vi "niDTS WLAN UTIL Freq to Channel.vi"(6 "secondary factor":i32(ring)=-1 items=["-1"=-1, "1"=1, "0"=0], 8 "error in":errorcluster, 9 "channel starting factor":dbl=10000.0, 10 "CH BW":T1=enum."160 MHz", 11 "Center Frequency":dbl) -> (0 "error out":errorcluster, 3 "Channel":u32)   [LabVIEW 2015, in "niDTS WLAN.lvlib"]
uses:
  niDTS WLAN.lvlib
  Includes/niDTS WLAN INC CH BW.ctl
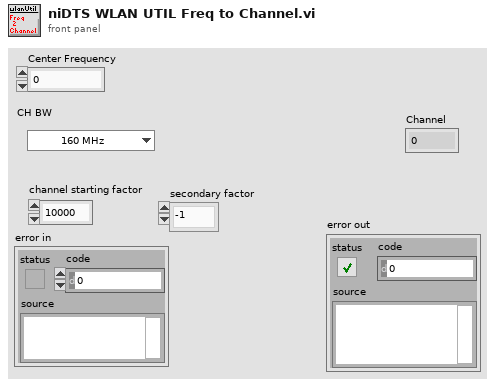
[diagram p1: front panel]
types:
  T1 = typedef "niDTS WLAN.lvlib/niDTS WLAN INC CH BW.ctl" = enum16{"20 MHz", "40 MHz", "80 MHz", "160 MHz"}
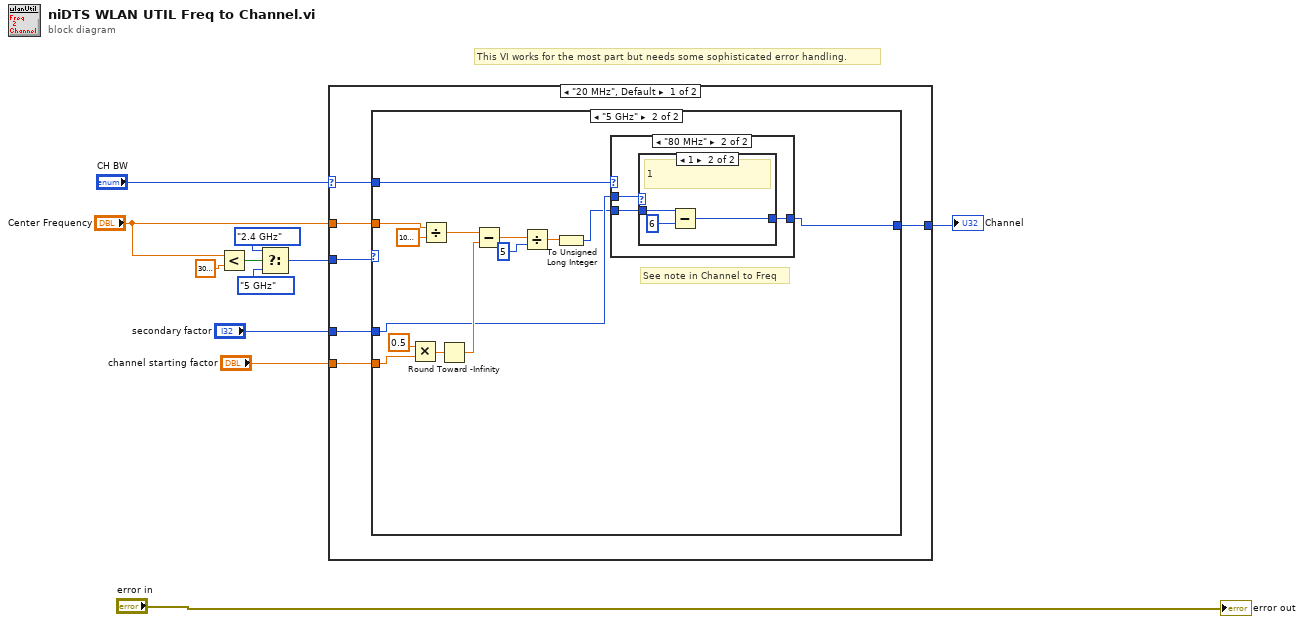
[diagram p0: block diagram]
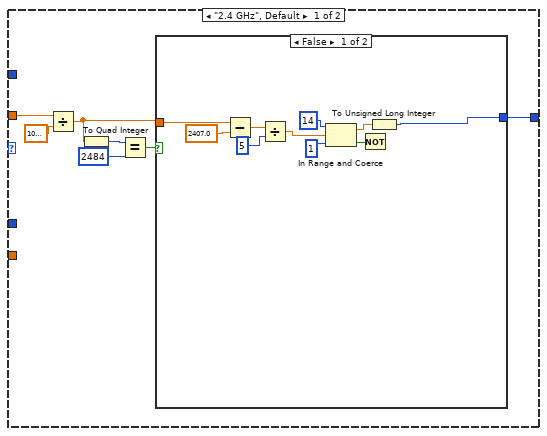
[diagram p2: hidden frame]
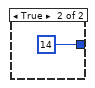
[diagram p3: hidden frame]
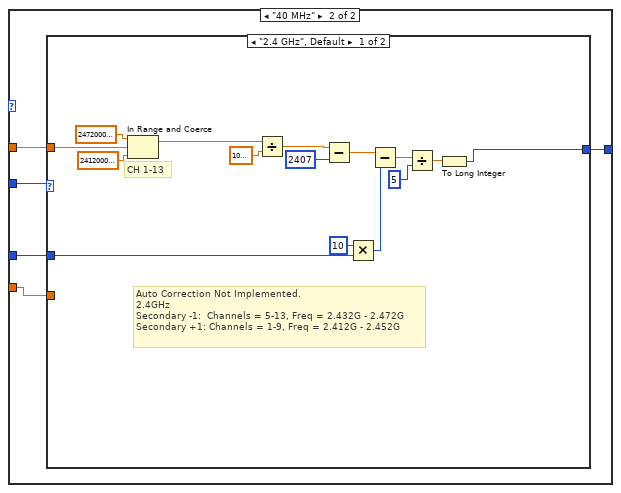
[diagram p6: hidden frame]
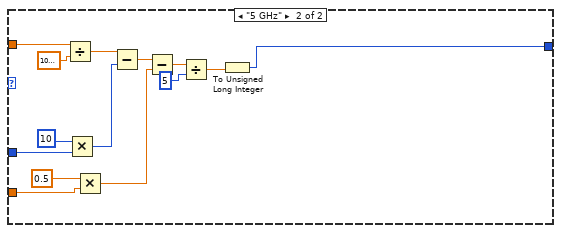
[diagram p7: hidden frame]
diagram:
  # "This VI works for the most part but needs some sophisticated error handling."
  n1 = Less?(x="Center Frequency", y=3000000000.0) -> (x < y?=w8:bool)
  n2 = Select(t=enum16{"2.4 GHz", "5 GHz"}."2.4 GHz" ("frequency band"), s=w8, f=enum16{"2.4 GHz", "5 GHz"}."5 GHz" ("frequency band")) -> (s? t:f=w7:enum16{"2.4 GHz", "5 GHz"})
  n3 = case shown="\"20 MHz\", Default" "CH BW" {
    selector: "CH BW" -> [w13 _]
    tunnel: w7 -> [w17 w62]
    tunnel: "Center Frequency" -> [w16 w61]
    tunnel: [w15 w59] -> w5
    tunnel: "secondary factor" -> [w12 w60]
    tunnel: "channel starting factor" -> [w14 w58]
    frame "20 MHz", Default {
      n4 = case shown="\"5 GHz\"" w17 {
        tunnel: w16 -> [w18 w40]
        tunnel: [w20 w36] -> w15
        tunnel: w14 -> [_ w45]
        tunnel: w13 -> [_ w39]
        tunnel: w12 -> [_ w38]
        frame "2.4 GHz", Default {
          n5 = Divide(x=w18, y=1000000.0) -> (x/y=w19:dbl)
          n6 = To Quad Integer(1:w19) -> (0:w23:i64)
          n7 = Equal?(x=w23, y=i64 2484) -> (x = y?=w21:bool)
          n8 = case shown="False" w21 {
            tunnel: [w25 u32 14 ("Channel")] -> w20
            tunnel: w19 -> [w33 _]
            frame False {
              n9 = Subtract(x=w33, y=2407.0 ("x")) -> (x-y=w32:dbl)
              n10 = Divide(x=w32, y=5) -> (x/y=w27:dbl)
              n11 = In Range and Coerce(upper limit=14, x=w27, lower limit=1) -> (coerced(x)=w26:dbl, In Range?=w30:bool)
              n12 = Not(x=w30) -> ()  [unwired: 1 out]
              n13 = To Unsigned Long Integer(number=w26) -> (unsigned 32bit integer=w25:u32)
            }
            frame True {
            }
          }
        }
        frame "5 GHz" {
          # "See note in Channel to Freq"
          n14 = Multiply(x=0.5, y=w45) -> (x*y=w47:dbl)
          n15 = Divide(x=w40, y=1000000.0) -> (x/y=w48:dbl)
          n16 = Round Toward -Infinity(1:w47) -> (0:w44:dbl)
          n17 = Subtract(x=w48, y=w44) -> (x-y=w43:dbl)
          n18 = Divide(x=w43, y=5) -> (x/y=w41:dbl)
          n19 = To Unsigned Long Integer(number=w41) -> (unsigned 32bit integer=w37:u32)
          n20 = case shown="\"80 MHz\"" w39 {
            tunnel: w38 -> [_ w53]
            tunnel: w37 -> [w50 w52]
            tunnel: [w50 w51] -> w36
            frame "20 MHz", Default {
            }
            frame "80 MHz" {
              n21 = case shown="1" w53 {
                tunnel: w52 -> [w54 w57]
                tunnel: [w54 w55] -> w51
                frame 0, Default {
                  # "-1 or 0"
                }
                frame 1 {
                  # "1"
                  n22 = Subtract(x=w57, y=6) -> (x-y=w55:u32)
                }
              }
            }
          }
        }
      }
    }
    frame "40 MHz" {
      n23 = case shown="\"2.4 GHz\", Default" w62 {
        tunnel: w61 -> [w75 w86]
        tunnel: w60 -> [w63 w88]
        tunnel: [w64 w78] -> w59
        tunnel: w58 -> [_ w90]
        frame "2.4 GHz", Default {
          # "Auto Correction Not Implemented.\n2.4GHz\nSecondary -1:  Channels = 5-13, Freq = 2.432G - 2.472G\nSecondary +1: Channels = 1-9, Freq = 2.412G - 2.452G"
          # "CH 1-13"
          n24 = In Range and Coerce(upper limit=2472000000.0 ("y"), x=w75, lower limit=2412000000.0 ("y")) -> (coerced(x)=w74:dbl)  [unwired: 1 out]
          n25 = Divide(x=w74, y=1000000.0) -> (x/y=w72:dbl)
          n26 = Subtract(x=w72, y=2407) -> (x-y=w70:dbl)
          n27 = Multiply(x=10, y=w63) -> (x*y=w68:i32)
          n28 = Subtract(x=w70, y=w68) -> (x-y=w67:dbl)
          n29 = Divide(x=w67, y=u32 5) -> (x/y=w65:dbl)
          n30 = To Long Integer(number=w65) -> (32bit integer=w64:i32)
        }
        frame "5 GHz" {
          n31 = Divide(x=w86, y=1000000.0) -> (x/y=w85:dbl)
          n32 = Multiply(x=10 ("y"), y=w88) -> (x*y=w84:i32)
          n33 = Multiply(x=0.5, y=w90) -> (x*y=w82:dbl)
          n34 = Subtract(x=w85, y=w84) -> (x-y=w83:dbl)
          n35 = Subtract(x=w83, y=w82) -> (x-y=w81:dbl)
          n36 = Divide(x=w81, y=5 ("x")) -> (x/y=w79:dbl)
          n37 = To Unsigned Long Integer(number=w79) -> (unsigned 32bit integer=w78:u32)
        }
      }
    }
  }
  "Channel" <- w5
  "error out" <- "error in"
